vi "ArrayWindow.VI"(9 "Index":i32, 10 "Total amount of Pts":i32, 11 "Input Y-values":dbl[](array[numeric])) -> (3 "Output Array":dbl[](array[numeric]))   [LabVIEW 2014]
panel:
  # "BufferArray.VI"
  # "Inputs"
  # "Outputs"
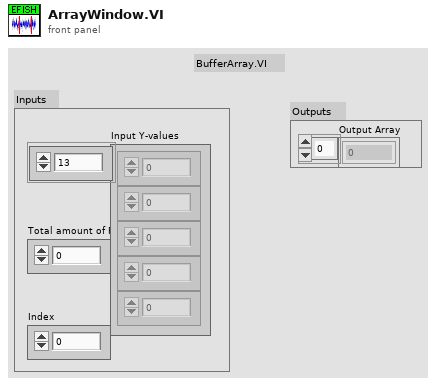
[diagram p1: front panel]
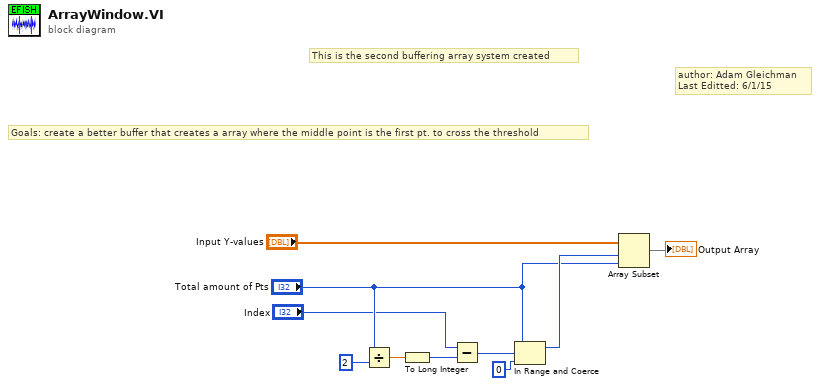
[diagram p0: block diagram]
diagram:
  # "author: Adam Gleichman\nLast Editted: 6/1/15"
  # "This is the second buffering array system created"
  # "Goals: create a better buffer that creates a array where the middle point is the first pt. to cross the threshold"
  n1 = Divide(x="Total amount of Pts", y=2) -> (x/y=w8:dbl)
  n2 = To Long Integer(number=w8) -> (32bit integer=w3:i32)
  n3 = Subtract(x="Index", y=w3) -> (x-y=w1:i32)
  n4 = In Range and Coerce(upper limit="Total amount of Pts", x=w1, lower limit=0) -> (coerced(x)=w6:i32)  [unwired: 1 out]
  n5 = Array Subset(array="Input Y-values", index=w6, length="Total amount of Pts") -> (→"Output Array":dbl[])
